vi "licdf verify genuine.vi"(0 "handle":i32, 1 "out_provisioned_date":string, 5 "out_genuine":i32, 7 "out_serial":string, 9 "serial_size":i32, 11 "error in (no error)":errorcluster, 12 "date_size":i32) -> (3 "out_provisioned_date out":string, 4 "function return":i32, 6 "out_genuine out":i32, 8 "out_serial out":string, 15 "error out":errorcluster)   [LabVIEW 2026, in "keynub_licdongle.lvlib"]
doc: "int32_t licdf_verify_genuine(int32_t handle, int32_t *out_genuine, char *out_serial,\n int32_t serial_size, char *out_provisioned_date,\n int32_t date_size);"
uses:
  keynub_licdongle.lvlib
  natives/win-x64/keynub_licdongle_flat.dll
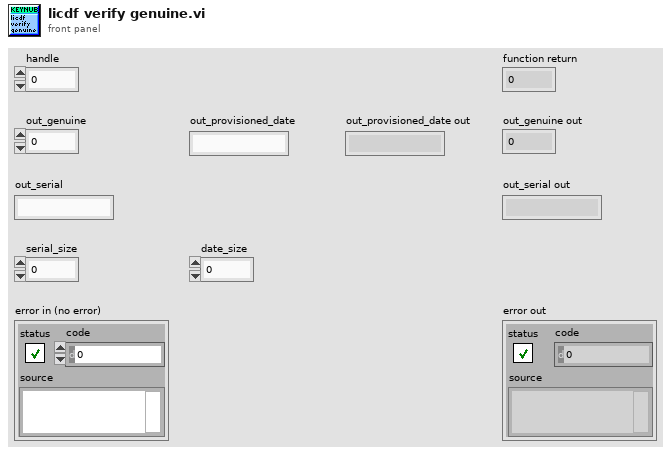
[diagram p1: front panel]
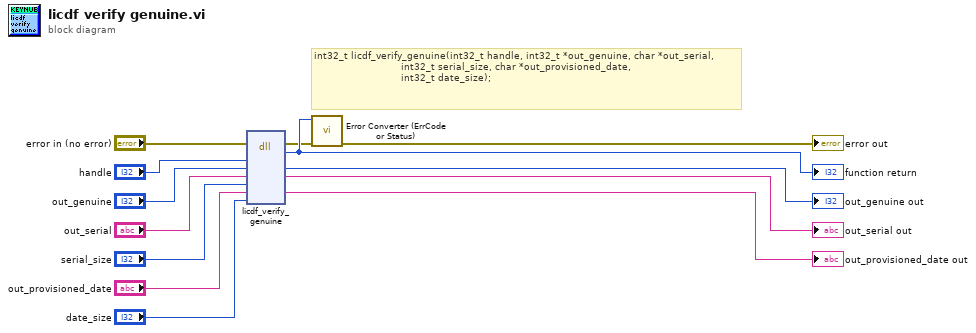
[diagram p0: block diagram]
diagram:
  # "int32_t licdf_verify_genuine(int32_t handle, int32_t *out_genuine, char *out_serial,\n                             int32_t serial_size, char *out_provisioned_date,\n                             int32_t date_size);"
  n1 = dll-call lib="C:/Austausch/KeyNub/LicenseDongle-PublicSDK/natives/win-x64/keynub_licdongle_flat.*" fn="licdf_verify_genuine"(error in="error in (no error)", "handle"="handle", "out_genuine"="out_genuine", "out_serial"="out_serial", "serial_size"="serial_size", "out_provisioned_date"="out_provisioned_date", "date_size"="date_size") -> (error out=w2:errorcluster, w13:i32, "out_genuine"=→"out_genuine out":i32, "out_serial"=→"out_serial out":string, "out_provisioned_date"=→"out_provisioned_date out":string)  [unwired: 5 in, 1 out]
  "function return" <- w13
  n2 = call "Error Converter (ErrCode or Status).vi"("error in (no error)"=w2, "error code"=w13) -> ("error out"=→"error out":errorcluster)  [unwired: 9 in]
